vi "Simple Read.vi"(4 "Abs_Waveform in":refnum<class "Abs_Waveform.lvclass">) -> (1 "Waveform":waveform(dbl))   [LabVIEW 2021, in "Abs_Waveform.lvclass"]
uses:
  Abs_Waveform.lvclass
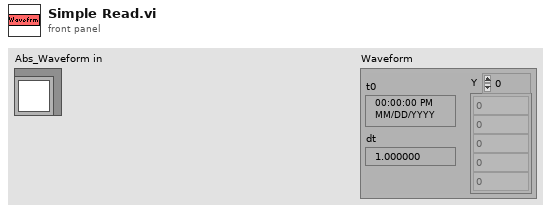
[diagram p1: front panel]
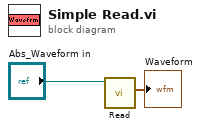
[diagram p0: block diagram]
diagram:
  n1 = call-dynamic "Read.vi"("Abs_Waveform in"="Abs_Waveform in") -> ("Waveform"=→"Waveform":waveform(dbl))  [unwired: 8 in, 2 out]
